vi "SC30_serial.vi"() -> ()   [LabVIEW 2009]
uses:
  <vilib>/Instr/_visa.llb/VISA Configure Serial Port (Instr).vi
panel:
  in  "Command":string
  out "bytes read":u32
  out "Response":string
  # "SC30 Serial Example"
  # "Enter command from the manual 5.7.5"
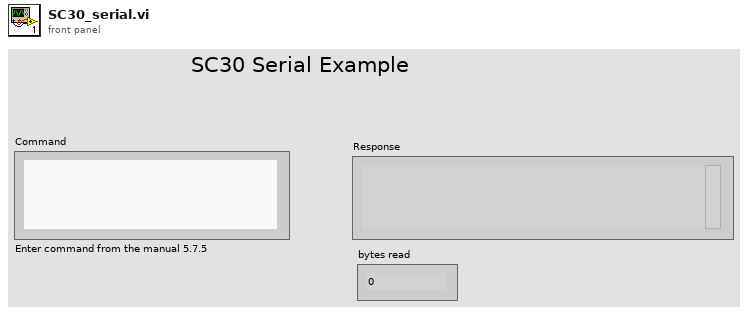
[diagram p1: front panel]
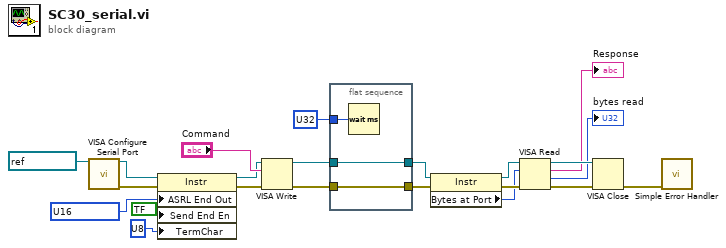
[diagram p0: block diagram]
diagram:
  w7 = u16 ? items=["None", "Last Bit", "TermChar", "Break"] ("Serial Settings:End Mode for Writes")
  n1 = call-poly "VISA Configure Serial Port"("VISA resource name"=refnum<visa-resource-name> ?) -> ("VISA resource name out"=w4:refnum<visa-resource-name>, "error out"=w2:errorcluster)  [unwired: 8 in, 5 out]
  n2 = property class="Instr"(reference=w4, error in=w2, "ASRL End Out"=w7, "Send End En"=bool ? ("Message Based Settings:Send End Enable"), "TermChar"=u8 ? ("Message Based Settings:Termination Character")) -> (reference out=w3:refnum<visa-resource-name>, error out=w1:errorcluster)
  n3 = VISA Write(VISA resource name=w3, write buffer="Command", error in (no error)=w1) -> (VISA resource name out=w14:refnum<visa-resource-name>, error out=w12:errorcluster)  [unwired: 1 out]
  n4 = flat-sequence {
    tunnel: u32 ? ("milliseconds to wait") -> [w23]
    tunnel: w14 -> [w25]
    tunnel: [w25] -> w13
    tunnel: w12 -> [w24]
    tunnel: [w24] -> w11
    frame #0 {
      n5 = Wait (ms)(milliseconds to wait=w23) -> ()  [unwired: 1 out]
    }
  }
  n6 = property class="Instr"(reference=w13, error in=w11) -> (reference out=w18:refnum<visa-resource-name>, error out=w19:errorcluster, "Bytes at Port"=w17:u32)
  n7 = VISA Read(VISA resource name=w18, byte count=w17, error in (no error)=w19) -> (VISA resource name out=w21:refnum<visa-resource-name>, read buffer=→"Response":string, return count=→"bytes read":u32, error out=w22:errorcluster)
  n8 = VISA Close(VISA resource name=w21, error in (no error)=w22) -> (error out=w10:errorcluster)
  n9 = call <vilib>:"Simple Error Handler.vi"("error in (no error)"=w10) -> ()  [unwired: 1 in, 8 out]
